vi "Get Client Rectangle.vi"(4 "error in (no error)":errorcluster, 7 "window refnum (NaWR)":T1) -> (0 "error out":errorcluster, 1 "window rect":T2, 3 "window refnum out":T1)   [LabVIEW 2023, in "WINUTIL.lvlib"]
doc: "This VI will find the coordinates of the upper left and lower right corners of the window identified by the 'window refnum' parameter. Coordinate values are in pixels, relative to the upper left corner of the screen. The 'window refnum' can be obtained by using 'Get Window RefNum.vi'."
uses:
  WINUTIL.lvlib
  Window Rectangle.ctl
  Window Refnum.ctl
  kernel32.dll
  user32.dll
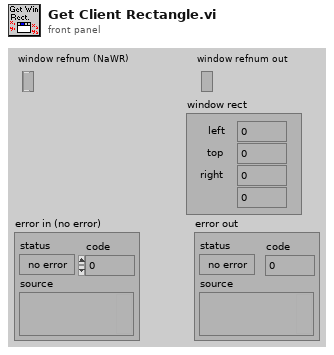
[diagram p1: front panel]
types:
  T1 = typedef "WINUTIL.lvlib/Window Refnum.ctl" = refnum<k1>
  T2 = typedef "WINUTIL.lvlib/Window Rectangle.ctl" = cluster{"left":i16, "top":i16, "right":i16, "bottom":i16}
  T3 = cluster{"RECT[0]":i32, "RECT[1]":i32, "RECT[2]":i32, "RECT[3]":i32}
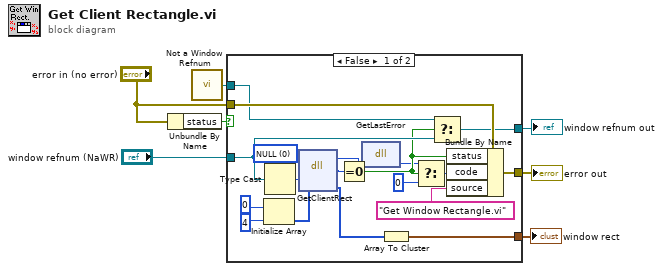
[diagram p0: block diagram]
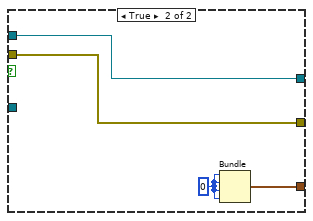
[diagram p2: hidden frame]
diagram:
  n1 = Unbundle By Name("error in (no error)") -> ("status"=w7:bool)
  n2 = call "Not a Window Refnum.vi"() -> ("Not a Window Refnum"=w3:T1)
  n3 = case shown="False" w7 {
    tunnel: "error in (no error)" -> [w24 w29]
    tunnel: [w23 w28] -> w2
    tunnel: [w22 w29] -> w5
    tunnel: "window refnum (NaWR)" -> [w19 _]
    tunnel: w3 -> [w18 w28]
    tunnel: [w11 w27] -> w1
    frame False {
      w20 = u32 0 items=["NULL"]
      n4 = Initialize Array(0, 4) -> (w15:i32[])
      n5 = Type Cast(type=w20, x=w19) -> (*(type *) &x=w21:u32)
      n6 = dll-call lib="USER32.DLL" fn="GetClientRect"("hWnd"=w21, "RECT"=w15) -> ("Return Value"=w9:i32, "RECT"=w12:i32[])  [unwired: 4 in, 2 out]
      n7 = Equal To 0?(x=w9) -> (x = 0?=w10:bool)
      n8 = dll-call lib="kernel32.dll" fn="GetLastError"(w9) -> (w8:i32)  [unwired: 2 in, 2 out]
      n9 = Array To Cluster(array=w12) -> (cluster=w11:T3)
      n10 = Select(t=w8, s=w10, f=0) -> (s? t:f=w14:i32)
      n11 = Select(t=w18, s=w10, f=w19) -> (s? t:f=w23:T1)
      n12 = Bundle By Name(cluster=w24, "status"=w10, "code"=w14, "source"="Get Window Rectangle.vi") -> (w22:errorcluster)
    }
    frame True {
      w26 = i16 0
      n13 = Bundle(w26, w26, w26, w26) -> (w27:cluster{i16, i16, i16, i16})  [unwired: 1 out]
    }
  }
  "error out" <- w5
  "window refnum out" <- w2
  "window rect" <- w1
